vi "New Dynamic Dispatch VI.vi"(8 "error in (no error)":errorcluster, 10 "App Refnum":refnum<vi>, 11 "SubVI Refnum":refnum<vi>) -> (0 "error out":errorcluster, 3 "Dynamic Dispatch VI Type out":refnum<class "Dynamic Dispatch VI Type.lvclass">)   [LabVIEW 2020, in "Peek Window.lvlib" / "Dynamic Dispatch VI Type.lvclass"]
uses:
  Dynamic Dispatch VI Type.lvclass
  D:/Code/VI-Peek/source/Peek Window/VI Types/Standard VI Type/Standard VI Type.lvclass
  Dynamic Dispatch VI Type.lvclass/Dynamic Dispatch VI Type.ctl
  Standard VI Type/Standard VI Type.lvclass/Standard VI Type.ctl
  Standard VI Type/Write App Refnum.vi
  Standard VI Type/Write VI Refnum.vi
  Standard VI Type/Write Full Qualified Name.vi
  Standard VI Type/Write Openable.vi
  Standard VI Type/Write Selectable.vi
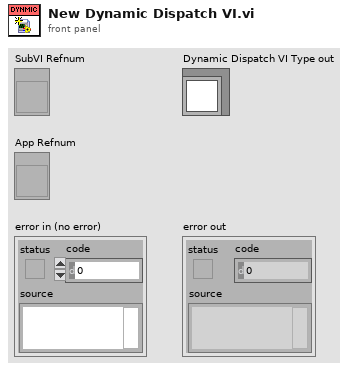
[diagram p1: front panel]
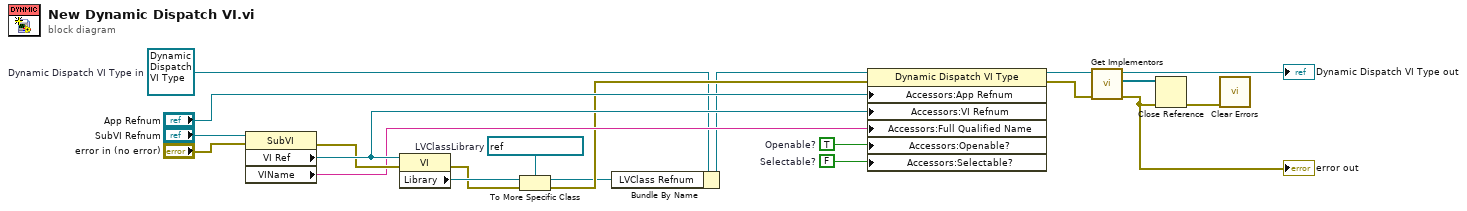
[diagram p0: block diagram]
diagram:
  w6 = FALSE  # Selectable?
  w7 = TRUE  # Openable?
  w17 = refnum<vi> refnum  # LVClassLibrary
  w3 = refnum<class "Dynamic Dispatch VI Type.lvclass"> refnum  # Dynamic Dispatch VI Type in
  n1 = property class="SubVI"(reference="SubVI Refnum", error in="error in (no error)") -> (error out=w19:errorcluster, "VI Ref"=w20:refnum<vi>, "VIName"=w18:string)  [unwired: 1 out]
  n2 = property class="VI"(reference=w20, error in=w19) -> (error out=w15:errorcluster, "Library"=w16:refnum<vi>)  [unwired: 1 out]
  n3 = To More Specific Class(target class=w17, reference=w16, error in=w15) -> (specific class reference=w1:refnum<vi>, error out=w8:errorcluster)
  n4 = Bundle By Name(cluster=w3, "LVClass Refnum"=w1) -> (w2:refnum<class "Dynamic Dispatch VI Type.lvclass">)
  n5 = property class="Dynamic Dispatch VI Type"(reference=w2, error in=w8, "Accessors:App Refnum"="App Refnum", "Accessors:VI Refnum"=w20, "Accessors:Full Qualified Name"=w18, "Accessors:Openable?"=w7, "Accessors:Selectable?"=w6) -> (reference out=w14:refnum<class "Dynamic Dispatch VI Type.lvclass">, error out=w9:errorcluster)
  n6 = call "Get Implementors.vi"("error in (no error)"=w9, "Dynamic Dispatch VI Type in"=w14) -> ("error out"=w10:errorcluster, "All Classes"=w12:refnum<vi>[], "Dynamic Dispatch VI Type out"=→"Dynamic Dispatch VI Type out":refnum<class "Dynamic Dispatch VI Type.lvclass">)  [unwired: 7 in]
  "error out" <- w10
  n7 = Close Reference(reference=w12, error in (no error)=w10) -> (error out=w11:errorcluster)
  n8 = call <vilib>:"Clear Errors.vi"("error in (no error)"=w11) -> ()  [unwired: 5 in, 2 out]
